vi "Update Configuration.vi"(8 "error in (no error)":errorcluster, 10 "FP Configuration":T1, 11 "reference in":refnum<class "Object.lvclass">) -> (0 "error out":errorcluster, 3 "reference out":refnum<class "Object.lvclass">)   [LabVIEW 2015, in "Front Panel Publisher.lvlib" / "Object.lvclass"]
uses:
  Object.lvclass
  Web Front Panel_class/Controls/FP Object Configuration.ctl
  Web Front Panel_class/Web Front Panel.lvclass
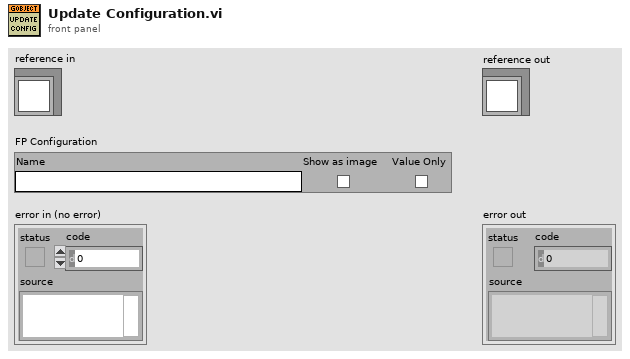
[diagram p1: front panel]
types:
  T1 = typedef "Front Panel Publisher.lvlib/Web Front Panel.lvclass/FP Object Configuration.ctl" = cluster{"Name":string, "Show as image":bool, "Value Only":bool}
  T2 = typedef "FrontPanelPublisher.lvlib/Object.lvclass/Attributes.ctl" = cluster{"UID":i32, "Type":string, "Coordinates":T3, "Reference":refnum<vi>}
  T3 = typedef "FrontPanelPublisher.lvlib/Object.lvclass/Coordinates.ctl" = cluster{"Left":i32, "Top":i32, "Height":u32, "Width":u32}
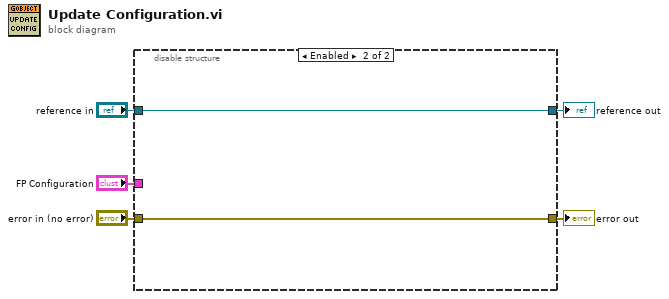
[diagram p0: block diagram]
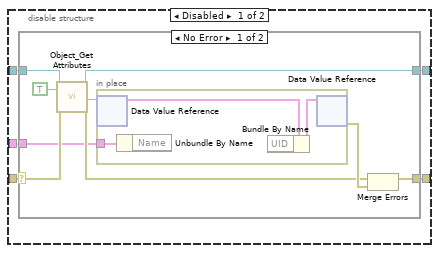
[diagram p2: hidden frame]
diagram:
  n1 = disable-structure shown="Enabled" {
    disable-tunnel: "error in (no error)" -> [w10 w26]
    disable-tunnel: [w9 w26] -> w4
    disable-tunnel: "reference in" -> [w8 w25]
    disable-tunnel: [w7 w25] -> w2
    disable-tunnel: "FP Configuration" -> [w6 _]
    frame Disabled {
      n2 = case shown="No Error" w10 {
        selector: w10 -> [w15 w24]
        tunnel: [w18 w24] -> w9
        tunnel: [w16 w23] -> w7
        tunnel: w8 -> [w17 w23]
        tunnel: w6 -> [w11 _]
        frame No Error {
          n3 = call "Object_Get Attributes.vi"("reference in"=w17, "OnlyGetDvrReference(False)"=TRUE, "error in (no error)"=w15) -> ("reference out"=w16:refnum<class "Object.lvclass">, "DataRef"=w14:refnum<data-value>, "error out"=w12:errorcluster)  [unwired: 13 in, 1 out]
          n4 = in-place {
            in-place-border: w11 -> [w20]
            n5 = in-place-dvr #1(w14) -> (w21:T2)  [unwired: 1 out]
            n6 = Unbundle By Name(w20) -> ()  [unwired: 1 out]
            n7 = Bundle By Name(cluster=w21) -> (w22:T2)  [unwired: 1 in]
            n8 = in-place-dvr #1(w22) -> (w19:errorcluster)  [unwired: 1 out]
          }
          n9 = Merge Errors(w12, w19) -> (w18:errorcluster)
        }
        frame Error {
        }
      }
    }
    frame Enabled {
    }
  }
  "error out" <- w4
  "reference out" <- w2
